vi "Low-Level Stream to Text File (NChan 1Samp).vi"() -> ()   [LabVIEW 2019]
uses:
  <vilib>/DAQmx/read.llb/DAQmx Read (Analog 1D DBL NChan 1Samp).vi
  <vilib>/DAQmx/create/channels.llb/DAQmx Create Channel (AI-Voltage-Basic).vi
  <vilib>/DAQmx/configure/timing.llb/DAQmx Timing (Sample Clock).vi
  <vilib>/DAQmx/miscellaneous.llb/DAQmx Fill In Error Info.vi
panel:
  in  "stop":bool
  out "Waveform Chart":T1(graph)
  in  "minimum value":dbl=-5.0
  in  "maximum value":dbl=5.0
  in  "Physical Channels":tag="PCI-6221/ai0:3"
  # "Measurement Range"
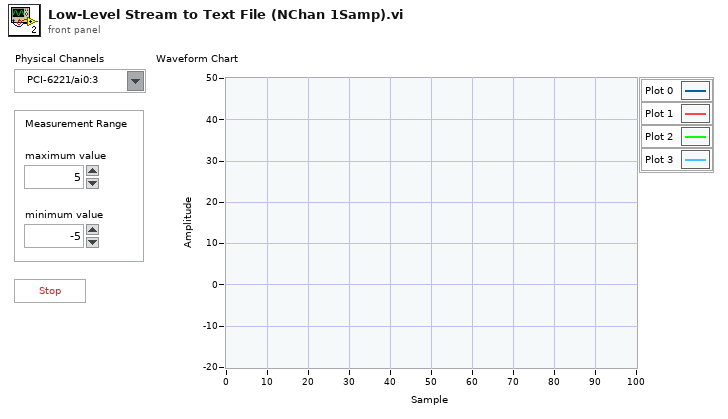
[diagram p1: front panel]
types:
  T1 = cluster{"data[0]":dbl, "data[1]":dbl, "data[2]":dbl, "data[3]":dbl, "data[4]":dbl, "data[5]":dbl, "data[6]":dbl, "data[7]":dbl, "data[8]":dbl}
  T2 = enum16{"open", "replace", "create", "open or create", "replace or create", "replace or create with confirmation"}
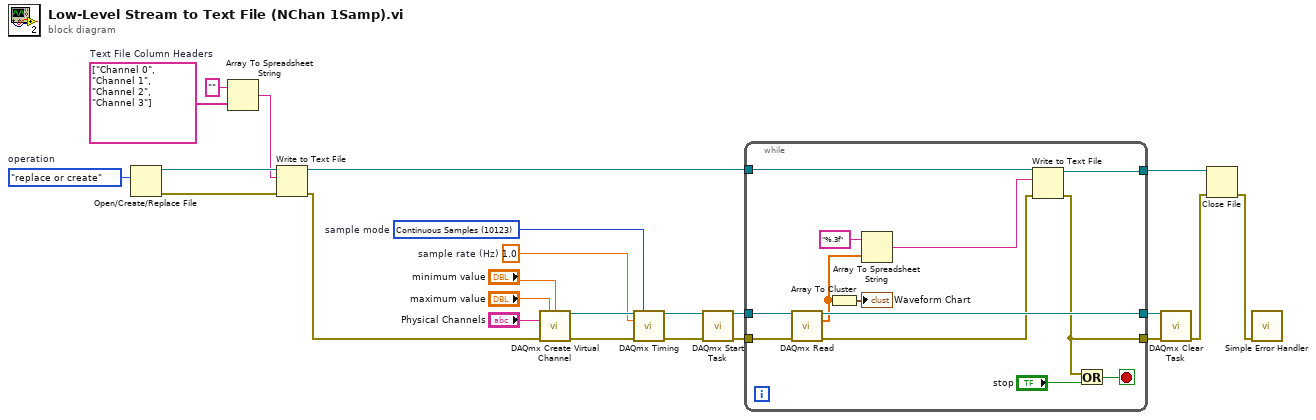
[diagram p0: block diagram]
diagram:
  w6 = string[] ["Channel 0", "Channel 1", "Channel 2", "Channel 3"]  # Text File Column Headers
  w10 = T2."replace or create"  # operation
  w19 = 1.0  # sample rate (Hz)
  w20 = 10123 items=["Finite Samples"=10178, "Continuous Samples"=10123, "Hardware Timed Single Point"=12522]  # sample mode
  n1 = Open/Create/Replace File(operation (0:open)=w10) -> (refnum out=w12:refnum<file>, error out=w11:errorcluster)  [unwired: 5 in, 1 out]
  n2 = Array To Spreadsheet String(array=w6, 3:"") -> (spreadsheet string=w5:string)  [unwired: 1 in]
  n3 = Write to Text File(file (use dialog)=w12, text=w5, error in=w11) -> (refnum out=w13:refnum<file>, error out=w14:errorcluster)  [unwired: 1 in, 1 out]
  n4 = call-poly <vilib>:"DAQmx Create Virtual Channel.vi"("maximum value"="maximum value", "minimum value"="minimum value", "physical channels"="Physical Channels", "error in"=w14) -> ("task out"=w24:refnum<k21>, "error out"=w23:errorcluster)  [unwired: 10 in]
  n5 = call-poly <vilib>:"DAQmx Timing.vi"("task/channels in"=w24, "sample mode"=w20, "rate"=w19, "error in"=w23) -> ("task out"=w18:refnum<k21>, "error out"=w17:errorcluster)  [unwired: 10 in]
  n6 = call <vilib>:"DAQmx Start Task.vi"("task/channels in"=w18, "error in"=w17) -> ("task out"=w22:refnum<k21>, "error out"=w21:errorcluster)  [unwired: 12 in]
  n7 = while {
    tunnel: w22 -> [w37]
    tunnel: w21 -> [w36]
    tunnel: [w35] -> w16
    tunnel: [w31] -> w15
    tunnel: w13 -> [w33]
    tunnel: [w32] -> w9
    stop <- w34 stop-if-true
    n8 = call-poly <vilib>:"DAQmx Read.vi"("task/channels in"=w37, "error in"=w36) -> ("task out"=w35:refnum<k21>, "data"=w29:dbl[], "error out"=w27:errorcluster)  [unwired: 11 in]
    n9 = Array To Cluster(array=w29) -> (cluster=→"Waveform Chart":T1)
    n10 = Array To Spreadsheet String(array=w29, 3:"%.3f" ("format string")) -> (spreadsheet string=w28:string)  [unwired: 1 in]
    n11 = Write to Text File(file (use dialog)=w33, text=w28, error in=w27) -> (refnum out=w32:refnum<file>, error out=w31:errorcluster)  [unwired: 1 in, 1 out]
    n12 = Or(x=w31, y="stop") -> (x .or. y?=w34:bool)
  }
  n13 = call <vilib>:"DAQmx Clear Task.vi"("task in"=w16, "error in"=w15) -> ("error out"=w8:errorcluster)  [unwired: 13 in]
  n14 = Close File(refnum=w9, error in=w8) -> (error out=w7:errorcluster)  [unwired: 1 out]
  n15 = call <vilib>:"Simple Error Handler.vi"("error in (no error)"=w7) -> ()  [unwired: 4 in, 5 out]
